vi "stateMachine3.vi"() -> ()   [LabVIEW 2020]
uses:
  C:/Users/DESKTOP-TLO0G68A/Desktop/LabVIEW/instrumentationLV/Thorlabs.MotionControl.Controls.dll
  Thorlabs.MotionControl.Controls.dll
  C:/Users/DESKTOP-TLO0G68A/Desktop/LabVIEW/instrumentationLV/ThorLabs.MotionControl.KCube.DCServoCLI.dll
  ThorLabs.MotionControl.KCube.DCServoCLI.dll
  C:/Users/DESKTOP-TLO0G68A/Desktop/LabVIEW/instrumentationLV/Thorlabs.MotionControl.GenericMotorCLI.dll
  Thorlabs.MotionControl.GenericMotorCLI.dll
  <instrlib>/Ocean Optics 2000 4000/Ocean Optics 2000 4000.lvlib
panel:
  out "Boolean 2":bool
  in  "initial y":dbl
  in  "initial x":dbl
  in  "save data":bool
  out "user selected path":path caption="selected path"
  out "pl background":dbl[](array[numeric])
  out "pl background signal":cluster{dbl[], dbl[]}(graph)
  in  "Enable Strobe (Disabled)":bool
  in  "spectrometer VISA":refnum<visa-resource-name>
  out "current y":i32
  out "current x":i32
  in  "y steps":i32
  in  "stepSize":dbl
  in  "x steps":i32
  in  "SerialNumber 2":string="27250520"
  in  "KCubeDCServoControl 2":refnum<k24>(container)
  in  "Begin Scan":bool
  in  "SerialNumber":string="27502753"
  in  "KCubeDCServoControl":refnum<k24>(container)
  # "You need to close the program completely before running a new scan."
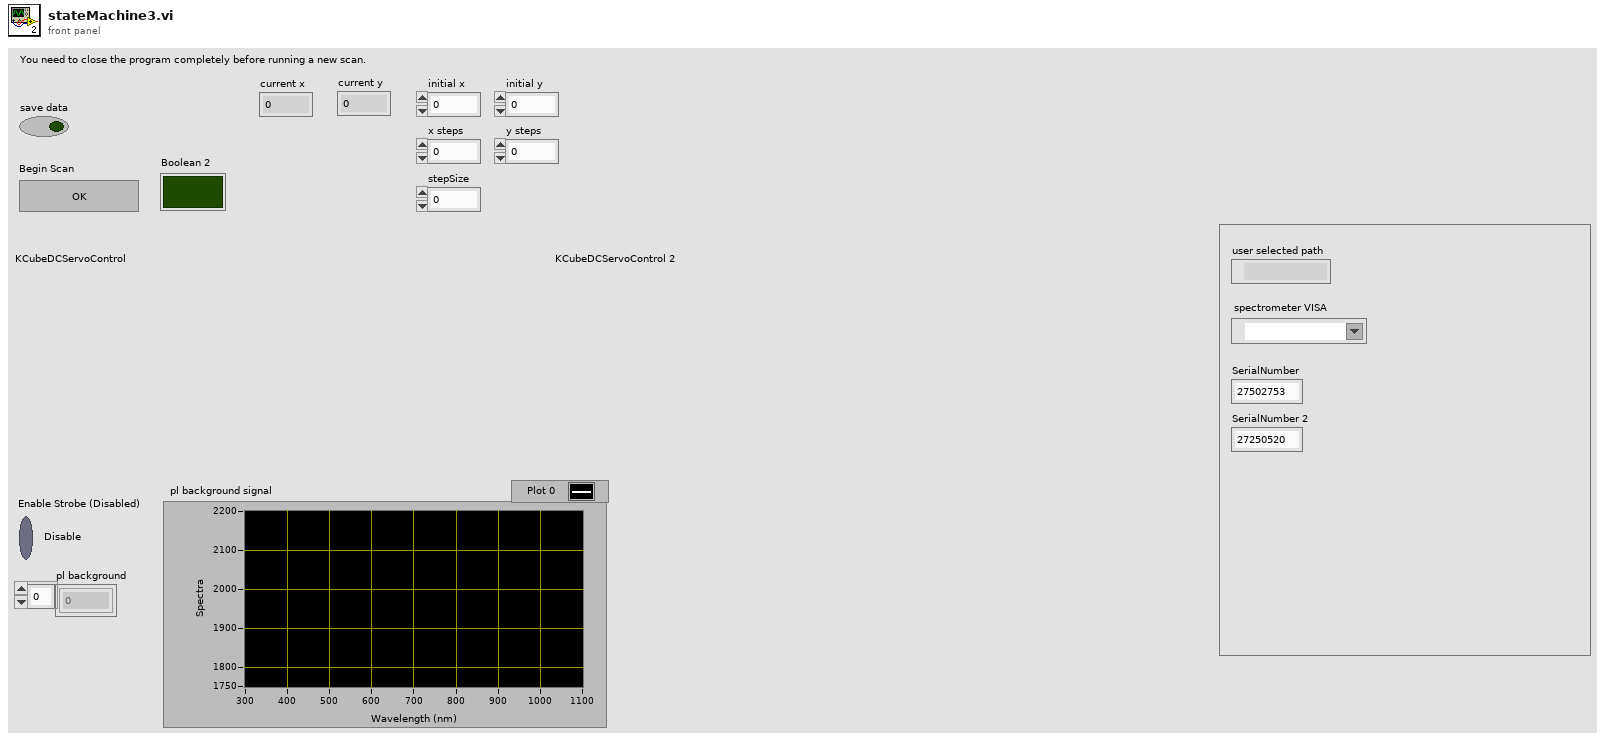
[diagram p1: front panel]
types:
  T1 = cluster{"Wavelength (nm)":dbl[], "Spectrum by Pixel Number":dbl[]}
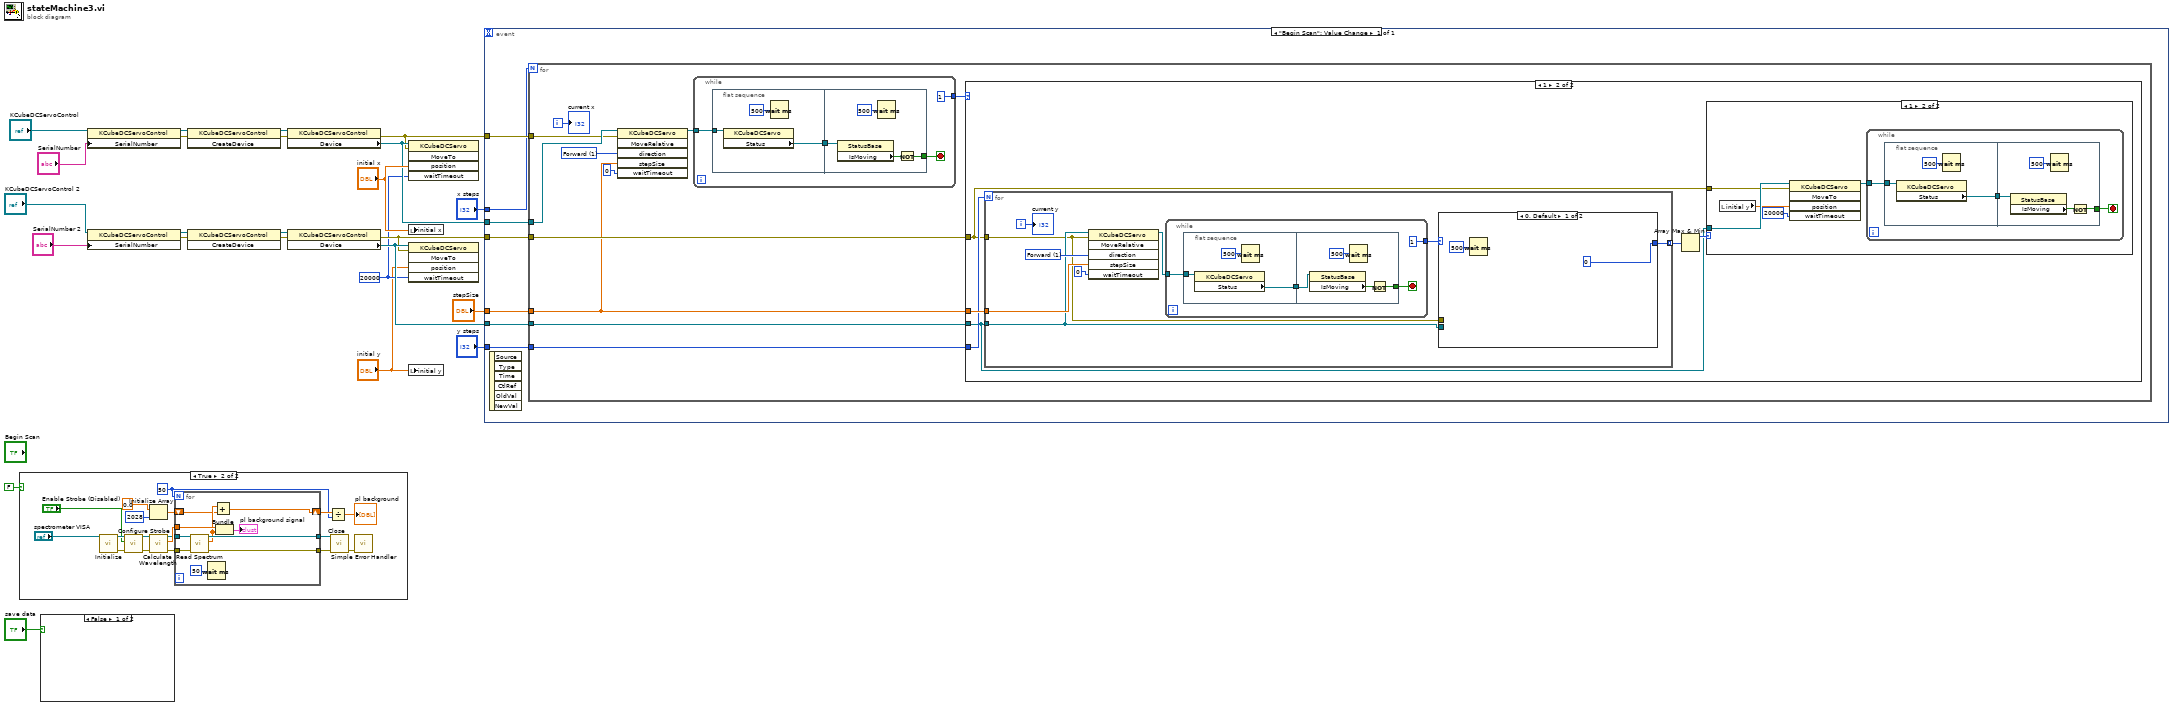
[diagram p0: block diagram]
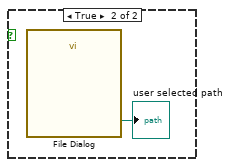
[diagram p3: hidden frame]
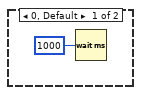
[diagram p4: hidden frame]
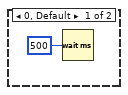
[diagram p5: hidden frame]
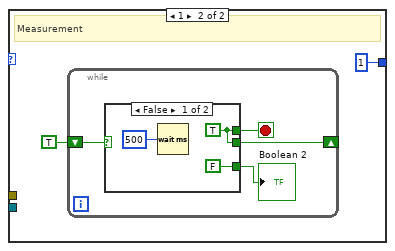
[diagram p6: hidden frame]
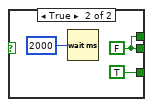
[diagram p7: hidden frame]
diagram:
  w3 = 20000 ("waitTimeout")
  n1 = case shown="True" FALSE {
    frame False {
    }
    frame True {
      w26 = 50
      n2 = call <instrlib>:"Initialize.vi"("VISA resource name"="spectrometer VISA") -> ("error out"=w41:errorcluster, "VISA resource name out"=w42:refnum<visa-resource-name>)  [unwired: 2 in, 7 out]
      n3 = call <instrlib>:"Configure Strobe.vi"("error in (no error)"=w41, "Enable Strobe (Disabled)"="Enable Strobe (Disabled)", "VISA resource name"=w42) -> ("error out"=w31:errorcluster, "VISA resource name out"=w32:refnum<visa-resource-name>)  [unwired: 7 out]
      n4 = call <instrlib>:"Calculate Wavelength.vi"("error in (no error)"=w31, "VISA resource name"=w32) -> ("error out"=w33:errorcluster, "Wavelength (nm)"=w35:dbl[], "VISA resource name out"=w34:refnum<visa-resource-name>)  [unwired: 1 in, 6 out]
      n5 = Initialize Array(0.0 ("element"), 2028 ("dimension size")) -> (w28:dbl[])
      n6 = for {
        N: w26 -> [_]
        tunnel: [w51] -> w39
        tunnel: [w50] -> w38
        tunnel: w35 -> [w49]
        tunnel: w34 -> [w48]
        tunnel: w33 -> [w47]
        shift-right: [w43] -> w27
        shift-left: w28 -> [w44]
        n7 = call <instrlib>:"Read Spectrum.vi"("error in (no error)"=w47, "VISA resource name"=w48) -> ("error out"=w50:errorcluster, "Spectrum by Pixel Number"=w45:dbl[], "VISA resource name out"=w51:refnum<visa-resource-name>)  [unwired: 6 in, 1 out]
        n8 = Wait (ms)(milliseconds to wait=u32 50 ("millisecond multiple")) -> ()  [unwired: 1 out]
        n9 = Add(x=w45, y=w44) -> (x+y=w43:dbl[])
        n10 = Bundle("Wavelength (nm)"=w49, "Spectrum by Pixel Number"=w45) -> (→"pl background signal":T1)  [unwired: 1 out]
      }
      n11 = Divide(x=w27, y=w26) -> (x/y=→"pl background":dbl[])
      n12 = call <instrlib>:"Close.vi"("error in (no error)"=w38, "VISA resource name"=w39) -> ("error out"=w37:errorcluster)  [unwired: 9 out]
      n13 = call <vilib>:"Simple Error Handler.vi"("error in (no error)"=w37) -> ()  [unwired: 1 in, 8 out]
    }
  }
  n14 = case shown="False" "save data" {
    frame False {
    }
    frame True {
      n15 = call "File Dialog"() -> ("selected path"=→"user selected path":path)  [unwired: 12 in, 3 out]
    }
  }
  n16 = property class="KCubeDCServoControl"(reference="KCubeDCServoControl", "SerialNumber"="SerialNumber") -> (reference out=w23:refnum<k24>, error out=w21:errorcluster)  [unwired: 1 in]
  n17 = property class="KCubeDCServoControl"(reference="KCubeDCServoControl 2", "SerialNumber"="SerialNumber 2") -> (reference out=w17:refnum<k24>, error out=w15:errorcluster)  [unwired: 1 in]
  n18 = invoke class="KCubeDCServoControl" method="CreateDevice"(reference=w23, error in=w21) -> (reference out=w22:refnum<k24>, error out=w20:errorcluster)  [unwired: 1 in, 1 out]
  n19 = invoke class="KCubeDCServoControl" method="CreateDevice"(reference=w17, error in=w15) -> (reference out=w16:refnum<k24>, error out=w14:errorcluster)  [unwired: 1 in, 1 out]
  n20 = property class="KCubeDCServoControl"(reference=w22, error in=w20) -> (error out=w6:errorcluster, "Device"=w7:refnum<k24>)  [unwired: 1 out]
  n21 = property class="KCubeDCServoControl"(reference=w16, error in=w14) -> (error out=w4:errorcluster, "Device"=w5:refnum<k24>)  [unwired: 1 out]
  n22 = invoke class="KCubeDCServo" method="MoveTo"(reference=w7, error in=w6, "position"="initial x", "waitTimeout"=w3) -> ()  [unwired: 1 in, 5 out]
  n23 = local write "initial x"("initial x") -> ()
  n24 = invoke class="KCubeDCServo" method="MoveTo"(reference=w5, error in=w4, "position"="initial y", "waitTimeout"=w3) -> ()  [unwired: 1 in, 5 out]
  n25 = local write "initial y"("initial y") -> ()
  n26 = event shown="[0] \"Begin Scan\": Value Change" {
    selector: _ -> [_]
    dyn-events: _ -> [_]
    timeout: _ -> [_]
    tunnel: w6 -> [w60]
    tunnel: w7 -> [w59]
    tunnel: w5 -> [w58]
    tunnel: w4 -> [w57]
    tunnel: "x steps" -> [w56]
    tunnel: "y steps" -> [w55]
    tunnel: "stepSize" -> [w54]
    event "Begin Scan": Value Change {
      n27 = event-data() -> ()  [unwired: 1 in, 6 out]
      n28 = for {
        N: w56 -> [_]
        tunnel: w54 -> [w61]
        tunnel: w59 -> [w64]
        tunnel: w60 -> [w63]
        tunnel: w55 -> [w71]
        tunnel: w58 -> [w70]
        tunnel: w57 -> [w69]
        i -> [w68]
        w67 = 1 items=["Forward"=1, "Backward"=2] ("direction")
        n29 = invoke class="KCubeDCServo" method="MoveRelative"(reference=w64, error in=w63, "direction"=w67, "stepSize"=w61, "waitTimeout"=0) -> (reference out=w65:refnum<k24>)  [unwired: 1 in, 5 out]
        n30 = while {
          tunnel: w65 -> [w74]
          tunnel: [1] -> w62
          stop <- w73 stop-if-true
          n31 = flat-sequence {
            tunnel: w74 -> [w78]
            tunnel: [w76] -> w75
            tunnel: [w79] -> w73
            tunnel: w75 -> [w81]
            frame #0 {
              n32 = property class="KCubeDCServo"(reference=w78) -> ("Status"=w76:refnum<k24>)  [unwired: 1 in, 2 out]
              n33 = Wait (ms)(milliseconds to wait=500) -> ()  [unwired: 1 out]
            }
            frame #1 {
              n34 = property class="StatusBase"(reference=w81) -> ("IsMoving"=w80:bool)  [unwired: 1 in, 2 out]
              n35 = Wait (ms)(milliseconds to wait=500) -> ()  [unwired: 1 out]
              n36 = Not(x=w80) -> (.not. x?=w79:bool)
            }
          }
        }
        n37 = case shown="1" w62 {
          tunnel: w61 -> [_ w89]
          tunnel: w71 -> [_ w88]
          tunnel: w70 -> [_ w85]
          tunnel: w69 -> [_ w84]
          frame 0, Default {
            n38 = Wait (ms)(milliseconds to wait=u32 1000) -> ()  [unwired: 1 out]
          }
          frame 1 {
            n39 = for {
              N: w88 -> [_]
              tunnel: w89 -> [w114]
              tunnel: w85 -> [w108]
              tunnel: w84 -> [w107]
              tunnel: [w106] -> w87 mode=indexing
              i -> [w113]
              w112 = 1 items=["Forward"=1, "Backward"=2] ("direction")
              n40 = invoke class="KCubeDCServo" method="MoveRelative"(reference=w108, error in=w107, "direction"=w112, "stepSize"=w114, "waitTimeout"=0) -> (reference out=w110:refnum<k24>)  [unwired: 1 in, 5 out]
              n41 = while {
                tunnel: w110 -> [w131]
                tunnel: [1] -> w109
                stop <- w130 stop-if-true
                n42 = flat-sequence {
                  tunnel: w131 -> [w135]
                  tunnel: [w133] -> w132
                  tunnel: w132 -> [w138]
                  tunnel: [w136] -> w130
                  frame #0 {
                    n43 = property class="KCubeDCServo"(reference=w135) -> ("Status"=w133:refnum<k24>)  [unwired: 1 in, 2 out]
                    n44 = Wait (ms)(milliseconds to wait=500) -> ()  [unwired: 1 out]
                  }
                  frame #1 {
                    n45 = property class="StatusBase"(reference=w138) -> ("IsMoving"=w137:bool)  [unwired: 1 in, 2 out]
                    n46 = Wait (ms)(milliseconds to wait=500) -> ()  [unwired: 1 out]
                    n47 = Not(x=w137) -> (.not. x?=w136:bool)
                  }
                }
              }
              n48 = case shown="0, Default" w109 {
                tunnel: w108 -> [_ _]
                tunnel: w107 -> [_ _]
                tunnel: [0 1] -> w106
                frame 0, Default {
                  n49 = Wait (ms)(milliseconds to wait=u32 500) -> ()  [unwired: 1 out]
                }
                frame 1 {
                  # "Measurement"
                  n50 = while {
                    shift-right: [w120] -> _
                    shift-left: TRUE -> [w122]
                    stop <- w119 stop-if-true
                    n51 = case shown="False" w122 {
                      tunnel: [FALSE TRUE] -> w121
                      tunnel: [w124 w126] -> w120
                      tunnel: [w124 w126] -> w119
                      frame False {
                        w124 = TRUE
                        n52 = Wait (ms)(milliseconds to wait=u32 500) -> ()  [unwired: 1 out]
                      }
                      frame True {
                        w126 = FALSE
                        n53 = Wait (ms)(milliseconds to wait=u32 2000) -> ()  [unwired: 1 out]
                      }
                    }
                    "Boolean 2" <- w121
                  }
                }
              }
              "current y" <- w113
            }
            n54 = Array Max & Min(array=w87) -> (max value=w86:i32)  [unwired: 3 out]
            n55 = case shown="1" w86 {
              tunnel: w85 -> [_ w95]
              tunnel: w84 -> [_ w94]
              frame 0, Default {
                n56 = Wait (ms)(milliseconds to wait=u32 500) -> ()  [unwired: 1 out]
              }
              frame 1 {
                n57 = local read "initial y"() -> (w92:dbl)
                n58 = invoke class="KCubeDCServo" method="MoveTo"(reference=w95, error in=w94, "position"=w92, "waitTimeout"=20000) -> (reference out=w93:refnum<k24>)  [unwired: 1 in, 4 out]
                n59 = while {
                  tunnel: w93 -> [w97]
                  stop <- w96 stop-if-true
                  n60 = flat-sequence {
                    tunnel: w97 -> [w101]
                    tunnel: [w99] -> w98
                    tunnel: [w102] -> w96
                    tunnel: w98 -> [w104]
                    frame #0 {
                      n61 = property class="KCubeDCServo"(reference=w101) -> ("Status"=w99:refnum<k24>)  [unwired: 1 in, 2 out]
                      n62 = Wait (ms)(milliseconds to wait=500) -> ()  [unwired: 1 out]
                    }
                    frame #1 {
                      n63 = property class="StatusBase"(reference=w104) -> ("IsMoving"=w103:bool)  [unwired: 1 in, 2 out]
                      n64 = Wait (ms)(milliseconds to wait=500) -> ()  [unwired: 1 out]
                      n65 = Not(x=w103) -> (.not. x?=w102:bool)
                    }
                  }
                }
              }
            }
          }
        }
        "current x" <- w68
      }
    }
  }
